vi "CVT Init.vi"(8 "error in (no error)":errorcluster, 11 "Tag List":T1[](array[typedef])) -> (0 "error out":errorcluster)   [LabVIEW 2010]
uses:
  Current Value Table.lvlib
  _SubVIs/TypeDefs/cvt_Data Types.ctl
  _SubVIs/TypeDefs/cvt_Tag Configuration.ctl
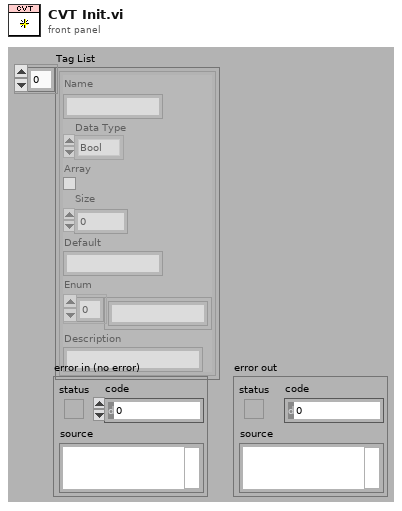
[diagram p1: front panel]
types:
  T1 = typedef "cvt_Tag Configuration.ctl" = cluster{"Name":string, "Data Type":T2, "Array":bool, "Size":u32, "Default":string, "Enum":string[], "Description":string}
  T2 = typedef "cvt_Data Types.ctl" = enum16{"Bool", "U8", "I32", "Double", "String", "Enum"}
  T3 = typedef "Current Value Table.lvlib/File Format.ctl" = cluster{"Tags":T4[], "Group Listings":T6[]}
  T4 = typedef "Current Value Table.lvlib/Single Tag.ctl" = cluster{"Data Type":T5, "Name":string, "Value":string, "Description":string}
  T5 = typedef "Current Value Table.lvlib/Data Types.ctl" = enum16{"Double", "Single", "I64", "I32", "I16", "I8", "U64", "U32", "U16", "U8", "String", "Boolean", "Array of U8", "Array of U16", "Array of U32", "Array of U64", "Array of I64", "Array of I32", "Array of I16", "Array of I8", "Array of Double", "Array of Single", "Array of Boolean", "Array of String"}
  T6 = typedef "Current Value Table.lvlib/Tag Grouping set.ctl" = cluster{"Group":string, "Tag Names":string[]}
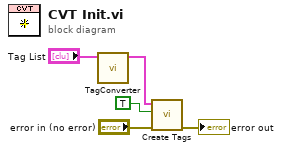
[diagram p0: block diagram]
diagram:
  n1 = call "TagConverter.vi"("CVT Tags"="Tag List") -> ("CVT Load Data"=w1:T3)  [unwired: 10 in]
  n2 = call "Create Tags.vi"("error in (no error)"="error in (no error)", "Clear Table? (F)"=TRUE ("Clear Engine?"), "CVT Tags to Create"=w1) -> ("error out"=→"error out":errorcluster)  [unwired: 8 in]
